vi "Configure Channels.vi"(8 "error in":errorcluster, 11 "DIO DO PWM DI Meas Freq CFG in":refnum<class "DIO DO PWM DI Meas Freq CFG.lvclass">) -> (0 "error out":errorcluster, 3 "DIO DO PWM DI Meas Freq CFG out":refnum<class "DIO DO PWM DI Meas Freq CFG.lvclass">)   [LabVIEW 2023, in "DIO DO PWM DI Meas Freq CFG.lvclass"]
uses:
  DIO DO PWM DI Meas Freq CFG.lvclass
  DIO DO PWM DI Meas Freq CFG.lvclass/DIO DO PWM DI Meas Freq CFG.ctl
  DO DAQmx Fixed Freq PWM CFG/DO DAQmx Fixed Freq PWM CFG.lvclass
  DI DAQmx CFG/DI DAQmx Meas Freq CFG.lvclass
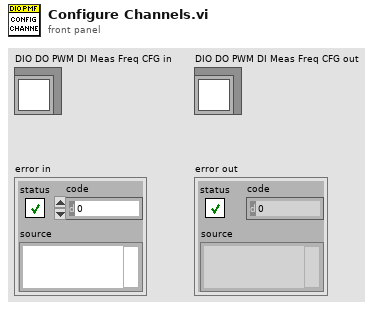
[diagram p1: front panel]
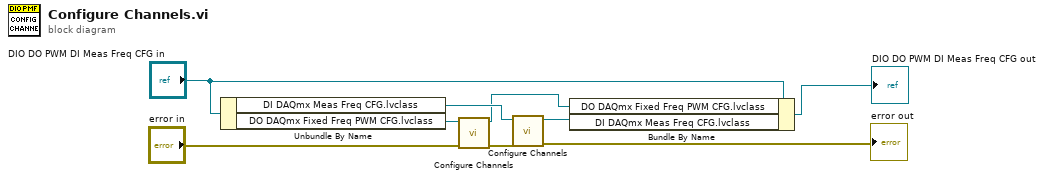
[diagram p0: block diagram]
diagram:
  n1 = Unbundle By Name("DIO DO PWM DI Meas Freq CFG in") -> ("DI DAQmx Meas Freq CFG.lvclass"=w6:refnum<class "DI DAQmx Meas Freq CFG.lvclass">, "DO DAQmx Fixed Freq PWM CFG.lvclass"=w9:refnum<class "DO DAQmx Fixed Freq PWM CFG.lvclass">)
  n2 = call-dynamic "Configure Channels.vi"("error in"="error in", "DO DAQmx Fixed Freq PWM CFG in"=w9) -> ("error out"=w7:errorcluster, "DO DAQmx Fixed Freq PWM CFG out"=w4:refnum<class "DO DAQmx Fixed Freq PWM CFG.lvclass">)  [unwired: 8 in]
  n3 = call-dynamic "Configure Channels.vi"("error in (no error)"=w7, "DI DAQmx CFG in"=w6) -> ("error out"=→"error out":errorcluster, "DI DAQmx CFG out"=w5:refnum<class "DI DAQmx Meas Freq CFG.lvclass">)  [unwired: 8 in]
  n4 = Bundle By Name(cluster="DIO DO PWM DI Meas Freq CFG in", "DO DAQmx Fixed Freq PWM CFG.lvclass"=w4, "DI DAQmx Meas Freq CFG.lvclass"=w5) -> (→"DIO DO PWM DI Meas Freq CFG out":refnum<class "DIO DO PWM DI Meas Freq CFG.lvclass">)
